vi "EEG_2021_099_Q1.vi"() -> ()   [LabVIEW 2022 SP3]
panel:
  out "result":dbl
  in  "c":dbl
  in  "b":dbl
  in  "a":dbl
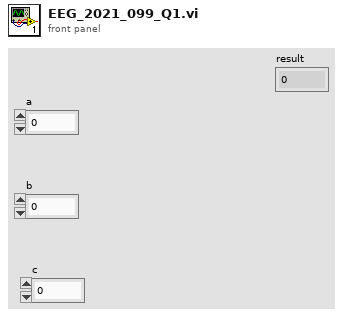
[diagram p1: front panel]
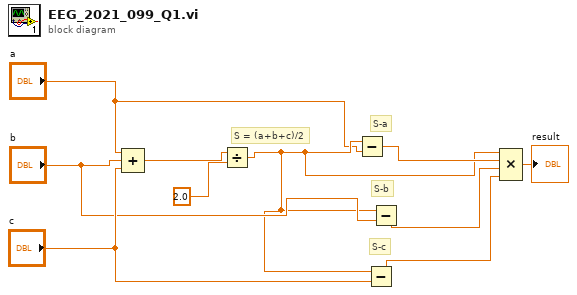
[diagram p0: block diagram]
diagram:
  # "S-c"
  # "S-b"
  # "S-a"
  # "S = (a+b+c)/2"
  n1 = Compound Arithmetic op=ADD("a", "b", "c") -> (w10:dbl)
  n2 = Divide(x=w10, y=2.0) -> (x/y=w2:dbl)
  n3 = Subtract(x=w2, y="a") -> (x-y=w6:dbl)
  n4 = Subtract(x=w2, y="c") -> (x-y=w4:dbl)
  n5 = Subtract(x=w2, y="b") -> (x-y=w5:dbl)
  n6 = Compound Arithmetic op=MULTIPLY(w2, w6, w5, w4) -> (→"result":dbl)
